vi "002 Parameter Set Control Name.vi"(8 "error in (no error)":errorcluster caption="Error In", 9 "Project":string, 10 "Read?":bool, 11 "Path In":path) -> (0 "error out":errorcluster caption="Error Out", 3 "Write":string[][](array[string]))   [LabVIEW 2020]
uses:
  0007 Controls/SY_Parameter.ctl
  Global/Data Global/Data Global Mode.ctl
  <vilib>/Utility/file.llb/Write Delimited Spreadsheet (string).vi
  <vilib>/Utility/file.llb/Read Delimited Spreadsheet (string).vi
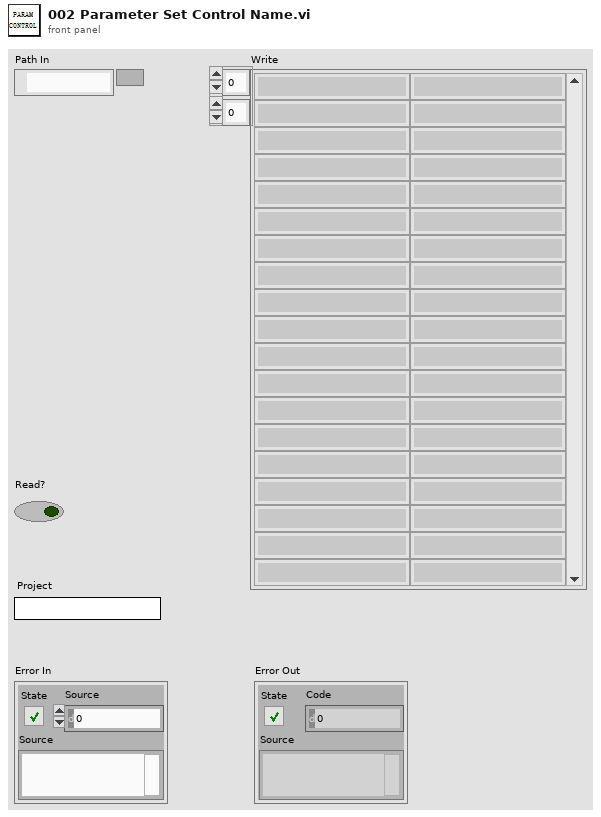
[diagram p1: front panel]
types:
  T1 = typedef "SY_Parameter.ctl" = cluster{"RH(%)":cluster{"DS":cluster{"阳极露点温度_DS":string, "阳极出口温度_DS":string, "阴极露点温度_DS":string, "阴极出口温度_DS":string, "阳极相对湿度_DS":string, "阴极相对湿度_DS":string, "阳极露点温度设置_DS":string, "阳极出口温度设置_DS":string, "阴极露点温度设置_DS":string, "阴极出口温度设置_DS":string}, "Value":cluster{"阳极露点温度_PV":sgl, "阳极出口温度_PV":sgl, "阴极露点温度_PV":sgl, "阴极出口温度_PV":sgl, "阳极相对湿度_SY":sgl, "阴极相对湿度_SY":sgl, "阳极露点温度设置_SV":sgl, "阳极出口温度设置_SV":sgl, "阴极露点温度设置_SV":sgl, "阴极出口温度设置_SV":sgl}}, "WEB":cluster{"DS":cluster{"自动模式(M0A1)_DS":string, "设备运行_DS":string, "工步号_DS":string, "运行模式_DS":string}, "Value":cluster{"自动模式(M0A1)_PV":bool, "设备运行_PV":bool, "工步号_PV":sgl, "运行模式_PV":bool}}, "ELD":cluster{"DS":cluster{"负载电压设置_DS":string, "负载电流设置_DS":string, "负载功率设置_DS":string, "负载模式设置_DS":string, "错误代码_DS":string, "负载电压_DS":string, "负载电流_DS":string, "负载功率_DS":string, "负载输出使能_DS":string, "负载连接_DS":string, "负载升压_DS":string, "负载升流_DS":string, "负载升功率_DS":string, "负载降压_DS":string, "负载降流_DS":string, "负载降功率_DS":string, "电流密度_DS":string, "功率密度_DS":string}, "Value":cluster{"负载电压设置_SV":sgl, "负载电流设置_SV":sgl, "负载功率设置_SV":sgl, "负载模式设置_SV":string, "错误代码_PV":string, "负载电压_PV":sgl, "负载电流_PV":sgl, "负载功率_PV":sgl, "负载输出使能_SV":bool, "负载连接_SY":bool, "负载升压_SV":sgl, "负载升流_SV":sgl, "负载升功率_SV":sgl, "负载降压_SV":sgl, "负载降流_SV":sgl, "负载降功率_SV":sgl, "电流密度_SV":sgl, "功率密度_SV":sgl}}, "SY":cluster{"DS":cluster{"总报警_DS":string, "WEB连接_DS":string, "计量比功能_DS":string, "PLC连接_DS":string, "H2计量比功能_DS":string, "Air计量比功能_DS":string, "PLC失联报警_DS":string}, "Value":cluster{"总报警_PV":bool, "WEB连接_PV":bool, "计量比功能_SV":bool, "PLC连接_SV":bool, "H2计量比功能_SV":bool, "Air计量比功能_SV":bool, "PLC失联报警_SV":bool}}, "PLC":cluster{"DS":cluster{"PLC急停_DS":string, "PLC连接_DS":string, "下位机心跳值_DS":string, "上位机心跳值_DS":string, "上位机报警等级字_DS":string, "负载可卸载_DS":string}, "Value":cluster{"PLC急停_PV":bool, "PLC连接_PV":bool, "下位机心跳值_PV":sgl, "上位机心跳值_SV":sgl, "上位机报警等级字_SV":sgl, "负载可卸载_SV":bool}}, "Bool Control":cluster{"DS":cluster{"维护模式_DS":string, "阳极氮气吹扫_DS":string, "阴极氮气吹扫_DS":string, "阳极脉冲使能_DS":string, "准备好使能_DS":string, "阳极干湿气切换_DS":string, "阴极干湿气切换_DS":string, "自动/手动模式_DS":string, "入口背压_DS":string, "手动卸载_DS":string, "软急停_DS":string, "负载连接_DS":string, "PLC故障复位_DS":string, "蜂鸣器屏蔽_DS":string}, "Value":cluster{"维护模式_SV":bool, "阳极氮气吹扫_SV":bool, "阴极氮气吹扫_SV":bool, "阳极脉冲使能_SV":bool, "准备好使能_SV":bool, "阳极干湿气切换_SV":bool, "阴极干湿气切换_SV":bool, "自动/手动模式_SV":bool, "入口背压_SV":bool, "手动卸载_SV":bool, "软急停_SV":bool, "负载连接_SV":bool, "PLC故障复位_SV":bool, "蜂鸣器屏蔽_SV":bool}}, "Stoich":cluster{"DS":cluster{"H2初始流量_DS":string, "Ait初始流量_DS":string, "H2侧系数_DS":string, "Air侧系数_DS":string, "H2计量比_DS":string, "Air计量比_DS":string, "时间间隔_DS":string, "H2计算气量_DS":string, "Air计算气量_DS":string, "H2流量_DS":string, "Air流量_DS":string}, "Value":cluster{"H2初始流量_SV":sgl, "Ait初始流量_SV":sgl, "H2侧系数_SV":sgl, "Air侧系数_SV":sgl, "H2计量比_SV":sgl, "Air计量比_SV":sgl, "时间间隔_SV":sgl, "H2计算气量_SV":sgl, "Air计算气量_SV":sgl, "H2流量_DS":sgl, "Air流量_DS":sgl}}, "PLC Need":cluster{"Name":string, "Identifier":string, "Source":string, "Value":string}[], "CVM":cluster{"DS":cluster{"活化面积_DS":string, "开路电压_DS":string, "单体总片数_DS":string, "单体显示片数_DS":string, "起始编号_DS":string, "最大值":string, "最大值编号_DS":string, "最小值_DS":string, "最小值编号_DS":string, "选区合计电压_DS":string, "平均值_DS":string, "离均差_DS":string}, "Value":cluster{"活化面积_SV":sgl, "开路电压_SV":sgl, "单体片数_SV":sgl, "单体显示片数_SV":sgl, "起始编号_SV":sgl, "最大值_SV":sgl, "最大值编号_SV":sgl, "最小值_SV":sgl, "最小值编号_SV":sgl, "选区合计电压_SV":sgl, "平均值_SV":sgl, "离均差_SV":sgl}}}
  T2 = typedef "Data Global Mode.ctl" = enum16{"Init", "Read", "Write", "Write Data", "Load"}
  T3 = cluster{"Name":string, "Identifier":string, "Source":string, "Value":string}[]
  T4 = cluster{"all rows[0]":string, "all rows[1]":string, "all rows[2]":string, "all rows[3]":string}
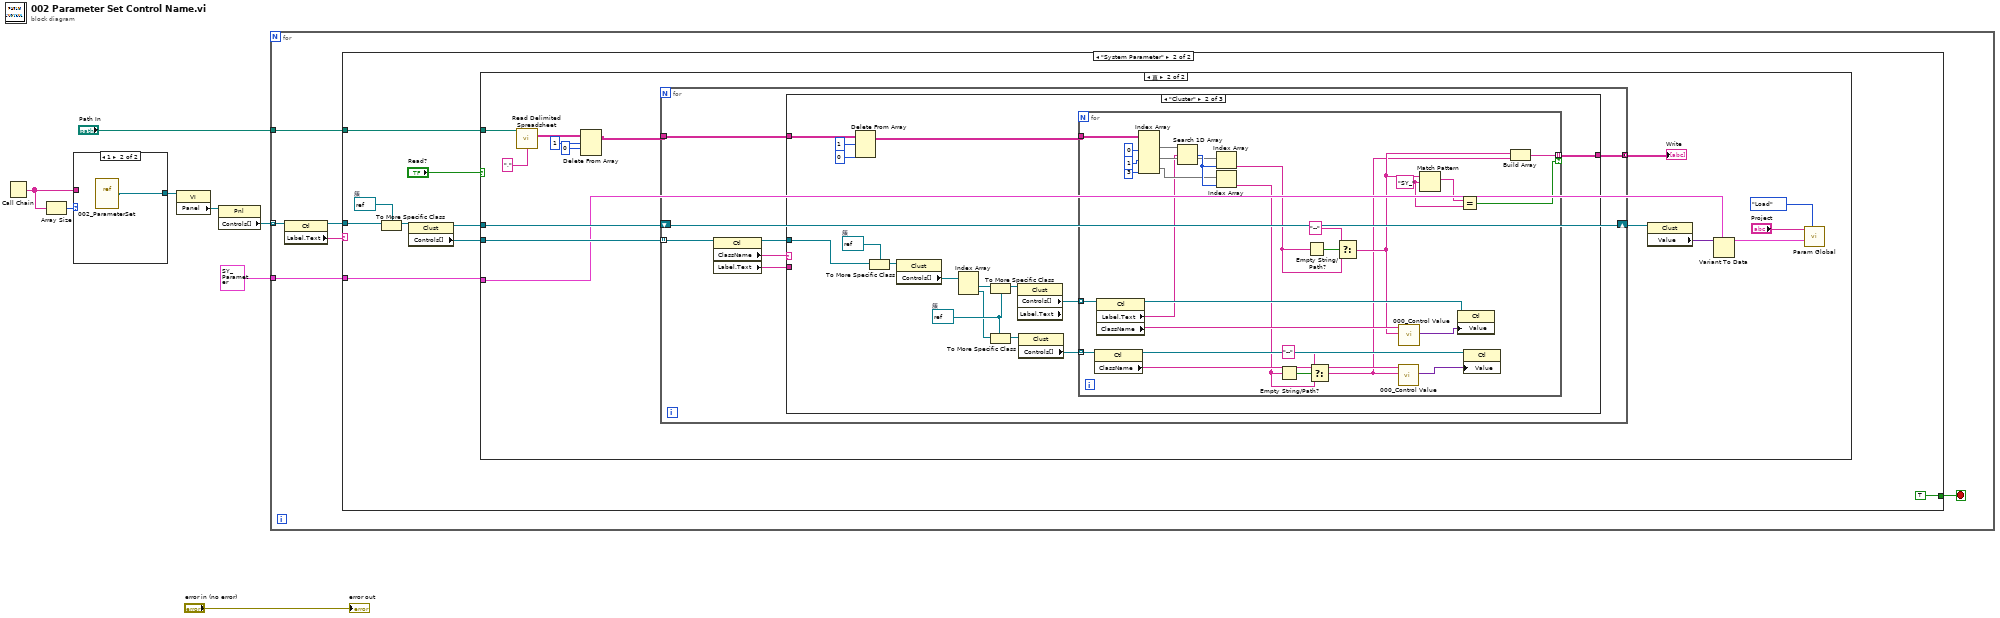
[diagram p0: block diagram]
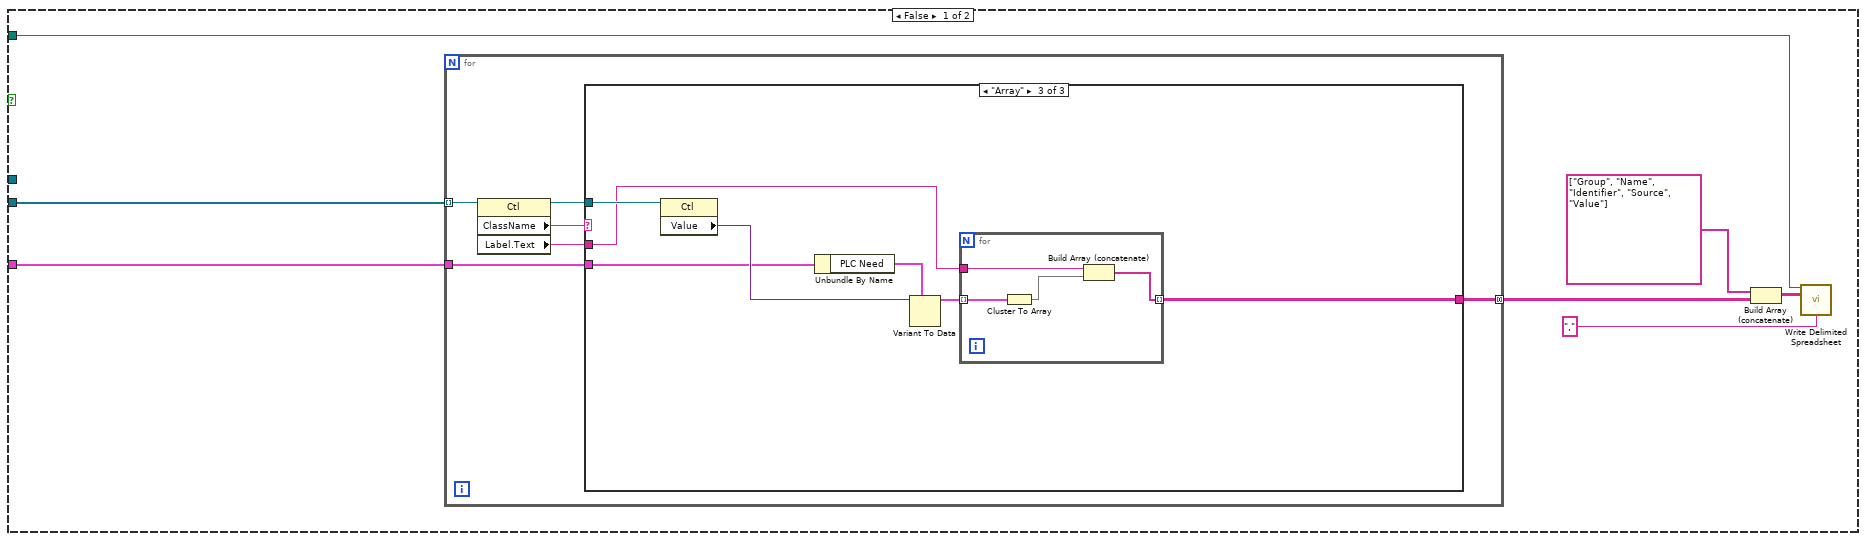
[diagram p3: hidden frame]
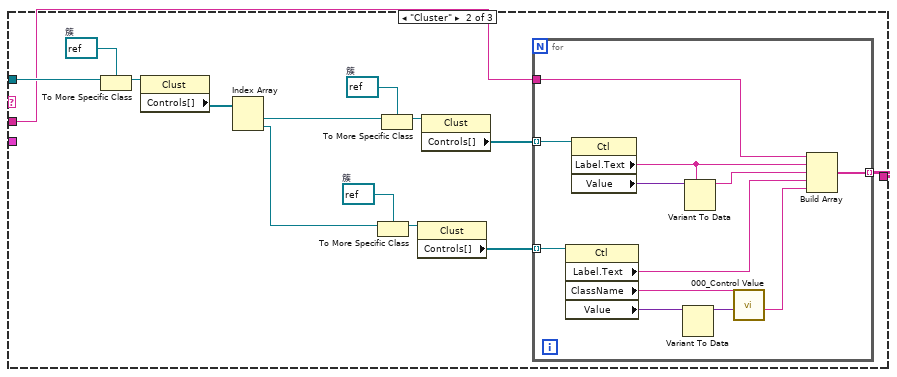
[diagram p5: hidden frame]
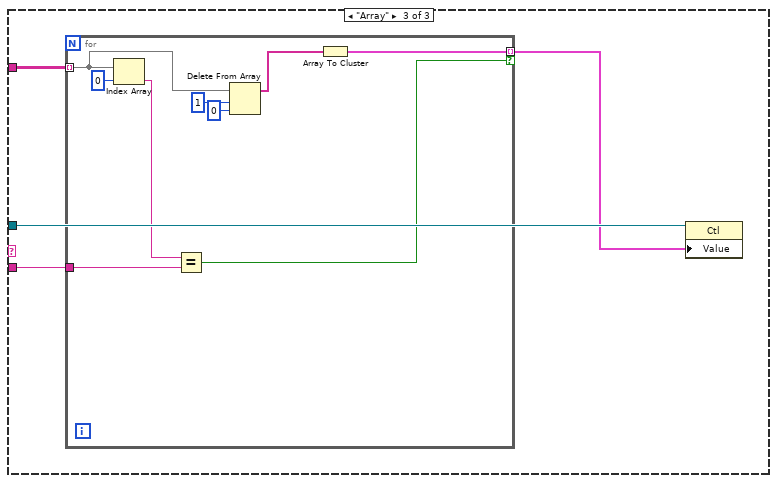
[diagram p7: hidden frame]
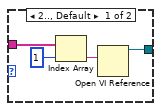
[diagram p8: hidden frame]
diagram:
  n1 = Call Chain() -> (call chain=w5:string[])
  n2 = Array Size(array=w5) -> (size(s)=w6:i32)
  n3 = case shown="1" w6 {
    tunnel: [w10 w13] -> w3
    tunnel: w5 -> [w9 _]
    frame 2.., Default {
      n4 = Index Array(array=w9, index=1 ("索引")) -> (element=w11:string)
      n5 = Open VI Reference(vi path=w11) -> (vi reference=w10:refnum<vi>)  [unwired: 5 in, 1 out]
    }
    frame 1 {
      n6 = vi-ref "002_ParameterSet.vi"() -> (w13:refnum<vi>)
    }
  }
  n7 = property class="VI"(reference=w3) -> ("Panel"=w4:refnum<vi>)  [unwired: 1 in, 2 out]
  n8 = property class="Pnl"(reference=w4) -> ("Controls[]"=w7:refnum<vi>[])  [unwired: 1 in, 2 out]
  n9 = for {
    tunnel: w7 -> [w19] mode=indexing
    tunnel: "Path In" -> [w15]
    tunnel: T1 {"RH(%)"={"DS"={"阳极露点温度_DS"="TIRC101_PV", "阳极出口温度_DS"="TIR104_PV", "阴极露点温度_DS"="TIRC301_PV", "阴极出口温度_DS"="TIRC301_PV", "阳极相对湿度_DS"="SY_RH_An", "阴极相对湿度_DS"="SY_RH_Ca", "阳极露点温度设置_DS"="TIRC101_PV", "阳极出口温度设置_DS"="TIR104_PV", "阴极露点温度设置_DS"="TIRC301_PV", "阴极出口温度设置_DS"="TIRC301_PV"}, "Value"={"阳极露点温度_PV"=0.0, "阳极出口温度_PV"=0.0, "阴极露点温度_PV"=0.0, "阴极出口温度_PV"=0.0, "阳极相对湿度_SY"=0.0, "阴极相对湿度_SY"=0.0, "阳极露点温度设置_SV"=0.0, "阳极出口温度设置_SV"=0.0, "阴极露点温度设置_SV"=0.0, "阴极出口温度设置_SV"=0.0}}, "WEB"={"DS"={"自动模式(M0A1)_DS"="AUTO_MODE", "设备运行_DS"="DEVICE_STATE", "工步号_DS"="DEVICE_STATE", "运行模式_DS"="DEVICE_STATE"}, "Value"={"自动模式(M0A1)_PV"=FALSE, "设备运行_PV"=FALSE, "工步号_PV"=0.0, "运行模式_PV"=FALSE}}, "ELD"={"DS"={"负载电压设置_DS"="EL_V_SET", "负载电流设置_DS"="EL_A_SET", "负载功率设置_DS"="EL_P_SET", "负载模式设置_DS"="EL_MODE", "错误代码_DS"="EL_ERROR", "负载电压_DS"="EL_V", "负载电流_DS"="EL_A", "负载功率_DS"="EL_P", "负载输出使能_DS"="EL_INPUT", "负载连接_DS"="ELD", "负载升压_DS"="SY_Load_Rise_Volt", "负载升流_DS"="SY_Load_Rise_Curr", "负载升功率_DS"="SY_Load_Rise_Power", "负载降压_DS"="SY_Load_Drop_Volt", "负载降流_DS"="SY_Load_Drop_Curr", "负载降功率_DS"="SY_Load_Drop_Power", "电流密度_DS"="Density_A_SV", "功率密度_DS"="Density_P_SV"}, "Value"={"负载电压设置_SV"=0.0, "负载电流设置_SV"=0.0, "负载功率设置_SV"=0.0, "负载模式设置_SV"="", "错误代码_PV"="", "负载电压_PV"=0.0, "负载电流_PV"=0.0, "负载功率_PV"=0.0, "负载输出使能_SV"=FALSE, "负载连接_SY"=FALSE, "负载升压_SV"=0.0, "负载升流_SV"=0.0, "负载升功率_SV"=0.0, "负载降压_SV"=0.0, "负载降流_SV"=0.0, "负载降功率_SV"=0.0, "电流密度_SV"=0.0, "功率密度_SV"=0.0}}, "SY"={"DS"={"总报警_DS"="SY_Totol_Warning", "WEB连接_DS"="SY_Web_Con", "计量比功能_DS"="SY_Measurung_Ratio", "PLC连接_DS"="SY_Measurung_Ratio", "H2计量比功能_DS"="SY_Measurung_Ratio", "Air计量比功能_DS"="SY_Measurung_Ratio", "PLC失联报警_DS"="SY_Measurung_Ratio"}, "Value"={"总报警_PV"=FALSE, "WEB连接_PV"=FALSE, "计量比功能_SV"=FALSE, "PLC连接_SV"=FALSE, "H2计量比功能_SV"=FALSE, "Air计量比功能_SV"=FALSE, "PLC失联报警_SV"=FALSE}}, "PLC"={"DS"={"PLC急停_DS"="HMI_Estop_SV", "PLC连接_DS"="PLC", "下位机心跳值_DS"="PLC", "上位机心跳值_DS"="HMI_AlarmWord_SV", "上位机报警等级字_DS"="HMI_AlarmWord_SV", "负载可卸载_DS"="HMI_AlarmWord_SV"}, "Value"={"PLC急停_PV"=FALSE, "PLC连接_PV"=FALSE, "下位机心跳值_PV"=0.0, "上位机心跳值_SV"=0.0, "上位机报警等级字_SV"=0.0, "负载可卸载_SV"=FALSE}}, "Bool Control"={"DS"={"维护模式_DS"="WorkMode_SV", "阳极氮气吹扫_DS"="An_Purge_SV", "阴极氮气吹扫_DS"="Ca_Purge_SV", "阳极脉冲使能_DS"="An_Pulse_EN_SV", "准备好使能_DS"="DEVICE_READY", "阳极干湿气切换_DS"="An_GasMode_SV", "阴极干湿气切换_DS"="Ca_GasMode_SV", "自动/手动模式_DS"="AUTO_MODE", "入口背压_DS"="Stack_PreMode_SV", "手动卸载_DS"="HMI_Stack_OFF_SV", "软急停_DS"="HMI_Estop_SV", "负载连接_DS"="ELoad_EN_SV", "PLC故障复位_DS"="PLC_Alarm_Reset_SV", "蜂鸣器屏蔽_DS"="BuzzerShield_SV"}, "Value"={"维护模式_SV"=FALSE, "阳极氮气吹扫_SV"=FALSE, "阴极氮气吹扫_SV"=FALSE, "阳极脉冲使能_SV"=FALSE, "准备好使能_SV"=FALSE, "阳极干湿气切换_SV"=FALSE, "阴极干湿气切换_SV"=FALSE, "自动/手动模式_SV"=FALSE, "入口背压_SV"=FALSE, "手动卸载_SV"=FALSE, "软急停_SV"=FALSE, "负载连接_SV"=FALSE, "PLC故障复位_SV"=FALSE, "蜂鸣器屏蔽_SV"=FALSE}}, "Stoich"={"DS"={"H2初始流量_DS"="SY_Activation_Area", "Ait初始流量_DS"="SY_Pieces", "H2侧系数_DS"="SY_Activation_Area", "Air侧系数_DS"="SY_Pieces", "H2计量比_DS"="SY_Activation_Area", "Air计量比_DS"="SY_Pieces", "时间间隔_DS"="SY_Stoich_Interval", "H2计算气量_DS"="SY_Stoich_H2Flow", "Air计算气量_DS"="SY_Stoich_AirFlow", "H2流量_DS"="SY_Stoich_H2Flow", "Air流量_DS"="SY_Stoich_AirFlow"}, "Value"={"H2初始流量_SV"=0.0, "Ait初始流量_SV"=0.0, "H2侧系数_SV"=0.0, "Air侧系数_SV"=0.0, "H2计量比_SV"=0.0, "Air计量比_SV"=0.0, "时间间隔_SV"=0.0, "H2计算气量_SV"=0.0, "Air计算气量_SV"=0.0, "H2流量_DS"=0.0, "Air流量_DS"=0.0}}, "PLC Need"=[], "CVM"={"DS"={"活化面积_DS"="SY_Activation_Area", "开路电压_DS"="SY_OCV_Value", "单体总片数_DS"="SY_Pieces", "单体显示片数_DS"="SY_Pieces_Dis", "起始编号_DS"="SY_Starting_Number", "最大值"="SY_Activation_Area", "最大值编号_DS"="SY_OCV_Value", "最小值_DS"="SY_Pieces", "最小值编号_DS"="SY_Pieces_Dis", "选区合计电压_DS"="SY_Starting_Number", "平均值_DS"="SY_Pieces_Dis", "离均差_DS"="SY_Starting_Number"}, "Value"={"活化面积_SV"=0.0, "开路电压_SV"=0.0, "单体片数_SV"=0.0, "单体显示片数_SV"=0.0, "起始编号_SV"=0.0, "最大值_SV"=0.0, "最大值编号_SV"=0.0, "最小值_SV"=0.0, "最小值编号_SV"=0.0, "选区合计电压_SV"=0.0, "平均值_SV"=0.0, "离均差_SV"=0.0}}} ("System Parameter") -> [w14]
    stop <- w16 stop-if-true
    n10 = property class="Ctl"(reference=w19) -> (reference out=w17:refnum<vi>, "Label.Text"=w18:string)  [unwired: 1 in, 1 out]
    n11 = case shown="\"System Parameter\"" w18 {
      tunnel: w17 -> [_ w27]
      tunnel: [_ TRUE] -> w16
      tunnel: w15 -> [_ w22]
      tunnel: w14 -> [_ w20]
      frame "eee", Default {
      }
      frame "System Parameter" {
        w26 = refnum<vi> refnum  # 簇
        n12 = To More Specific Class(target class=w26, reference=w27) -> (specific class reference=w25:refnum<vi>)  [unwired: 1 in, 1 out]
        n13 = property class="Clust"(reference=w25) -> (reference out=w21:refnum<vi>, "Controls[]"=w24:refnum<vi>[])  [unwired: 1 in, 1 out]
        n14 = case shown="真" "Read?" {
          tunnel: w24 -> [w35 w89]
          tunnel: w22 -> [w30 w93]
          tunnel: w21 -> [_ w88]
          tunnel: w20 -> [w31 w85]
          frame False {
            n15 = for {
              tunnel: w35 -> [w41] mode=indexing
              tunnel: [w37] -> w29 mode=concatenating
              tunnel: w31 -> [w36]
              n16 = property class="Ctl"(reference=w41) -> (reference out=w38:refnum<vi>, "ClassName"=w40:string, "Label.Text"=w39:string)  [unwired: 1 in, 1 out]
              n17 = case shown="\"Array\"" w40 {
                tunnel: w39 -> [_ w42 w69]
                tunnel: w38 -> [_ w54 w74]
                tunnel: [_ w51 w70] -> w37
                tunnel: w36 -> [_ _ w68]
                frame "eee", Default {
                }
                frame "Cluster" {
                  w47 = refnum<vi> refnum  # 簇
                  w49 = refnum<vi> refnum  # 簇
                  w55 = refnum<vi> refnum  # 簇
                  n18 = To More Specific Class(target class=w55, reference=w54) -> (specific class reference=w53:refnum<vi>)  [unwired: 1 in, 1 out]
                  n19 = property class="Clust"(reference=w53) -> ("Controls[]"=w52:refnum<vi>[])  [unwired: 1 in, 2 out]
                  n20 = Index Array(array=w52) -> (element #1=w48:refnum<vi>, element #2=w45:refnum<vi>)  [unwired: 2 in]
                  n21 = To More Specific Class(target class=w47, reference=w45) -> (specific class reference=w46:refnum<vi>)  [unwired: 1 in, 1 out]
                  n22 = To More Specific Class(target class=w49, reference=w48) -> (specific class reference=w50:refnum<vi>)  [unwired: 1 in, 1 out]
                  n23 = property class="Clust"(reference=w46) -> ("Controls[]"=w44:refnum<vi>[])  [unwired: 1 in, 2 out]
                  n24 = property class="Clust"(reference=w50) -> ("Controls[]"=w43:refnum<vi>[])  [unwired: 1 in, 2 out]
                  n25 = for {
                    tunnel: [w59] -> w51 mode=indexing
                    tunnel: w44 -> [w58] mode=indexing
                    tunnel: w43 -> [w57] mode=indexing
                    tunnel: w42 -> [w56]
                    n26 = property class="Ctl"(reference=w58) -> ("Label.Text"=w61:string, "ClassName"=w62:string, "Value"=w66:variant)  [unwired: 1 in, 2 out]
                    n27 = property class="Ctl"(reference=w57) -> ("Label.Text"=w65:string, "Value"=w67:variant)  [unwired: 1 in, 2 out]
                    n28 = Variant To Data(Variant=w66) -> (data=w63:variant)  [unwired: 2 in, 1 out]
                    n29 = Variant To Data(type=w65, Variant=w67) -> (data=w64:string)  [unwired: 1 in, 1 out]
                    n30 = call "000_Control Value.vi"("Value In"=w63, "Class Name"=w62) -> ("Value String Out"=w60:string)  [unwired: 8 in, 1 out]
                    n31 = Build Array(w56, w65, w64, w61, w60) -> (w59:string[])
                  }
                }
                frame "Array" {
                  n32 = property class="Ctl"(reference=w74) -> ("Value"=w72:variant)  [unwired: 1 in, 2 out]
                  n33 = Unbundle By Name(w68) -> ("PLC Need"=w73:T3)
                  n34 = Variant To Data(type=w73, Variant=w72) -> (data=w71:T3)  [unwired: 1 in, 1 out]
                  n35 = for {
                    tunnel: w71 -> [w78] mode=indexing
                    tunnel: [w76] -> w70 mode=indexing
                    tunnel: w69 -> [w75]
                    n36 = Cluster To Array(cluster=w78) -> (array=w77:string[])
                    n37 = Build Array (concatenate)(w75, w77) -> (w76:string[])
                  }
                }
              }
            }
            n38 = Build Array (concatenate)(string[] ["Group", "Name", "Identifier", "Source", "Value"], w29) -> (w33:string[][])
            n39 = call-poly <vilib>:"Write Delimited Spreadsheet.vi"("file path (dialog if empty)"=w30, "2D data"=w33, "delimiter (\\t)"="," ("delimiter (\\t)")) -> ()  [unwired: 11 in, 2 out]
          }
          frame True {
            n40 = call-poly <vilib>:"Read Delimited Spreadsheet.vi"("file path (dialog if empty)"=w93, "delimiter (\\t)"="," ("delimiter (\\t)")) -> ("all rows"=w83:string[][])  [unwired: 8 in, 5 out]
            n41 = Delete From Array(array=w83, length=1 ("长度"), index (row)=0 ("禁用的索引 (列)")) -> (array with subset deleted=w80:string[][])  [unwired: 1 in, 1 out]
            n42 = for {
              tunnel: w89 -> [w99] mode=indexing
              shift-right: [w100] -> w87
              shift-left: w88 -> [w100]
              tunnel: w80 -> [w98]
              tunnel: [w94] -> w79 mode=concatenating
              n43 = property class="Ctl"(reference=w99) -> (reference out=w97:refnum<vi>, "ClassName"=w96:string, "Label.Text"=w95:string)  [unwired: 1 in, 1 out]
              n44 = case shown="\"Cluster\"" w96 {
                tunnel: w98 -> [_ w103 w149]
                tunnel: w97 -> [_ w106 w147]
                tunnel: w95 -> [_ _ w148]
                tunnel: [_ w101 _] -> w94
                frame "eee", Default {
                }
                frame "Cluster" {
                  w109 = refnum<vi> refnum  # 簇
                  w108 = refnum<vi> refnum  # 簇
                  n45 = Delete From Array(array=w103, length=1 ("长度"), index (col)=0 ("禁用的索引 (列)")) -> (array with subset deleted=w102:string[][])  [unwired: 1 in, 1 out]
                  n46 = To More Specific Class(target class=w108, reference=w106) -> (specific class reference=w110:refnum<vi>)  [unwired: 1 in, 1 out]
                  n47 = property class="Clust"(reference=w110) -> ("Controls[]"=w111:refnum<vi>[])  [unwired: 1 in, 2 out]
                  n48 = Index Array(array=w111) -> (element #1=w115:refnum<vi>, element #2=w107:refnum<vi>)  [unwired: 2 in]
                  n49 = To More Specific Class(target class=w109, reference=w115) -> (specific class reference=w112:refnum<vi>)  [unwired: 1 in, 1 out]
                  n50 = To More Specific Class(target class=w109, reference=w107) -> (specific class reference=w114:refnum<vi>)  [unwired: 1 in, 1 out]
                  n51 = property class="Clust" props=["Controls[]", "Label", "Text"](reference=w112) -> ("Controls[]"=w113:refnum<vi>[])  [unwired: 1 in, 3 out]
                  n52 = property class="Clust"(reference=w114) -> ("Controls[]"=w116:refnum<vi>[])  [unwired: 1 in, 2 out]
                  n53 = for {
                    tunnel: w113 -> [w141] mode=indexing
                    tunnel: w116 -> [w145] mode=indexing
                    tunnel: w102 -> [w130]
                    tunnel: [w118] -> w101 mode=indexing if=w117
                    w121 = "SY_" ("正则表达式")
                    n54 = property class="Ctl"(reference=w145) -> (reference out=w143:refnum<vi>, "ClassName"=w144:string)  [unwired: 1 in, 1 out]
                    n55 = property class="Ctl"(reference=w141) -> (reference out=w138:refnum<vi>, "Label.Text"=w123:string, "ClassName"=w140:string)  [unwired: 1 in, 1 out]
                    n56 = Index Array(array=w130, index (col) #1=0 ("禁用的索引 (列)"), index (col) #2=1 ("索引 (列)"), index (col) #3=3 ("索引 (列)")) -> (element #1=w134:string[], element #2=w135:string[], element #3=w136:string[])  [unwired: 3 in]
                    n57 = Search 1D Array(1D array=w134, element=w123) -> (index of element=w137:i32)  [unwired: 1 in]
                    n58 = Index Array(array=w135, index=w137) -> (element=w124:string)
                    n59 = Index Array(array=w136, index=w137) -> (element=w127:string)
                    n60 = Empty String/Path?(string/path=w127) -> (empty?=w129:bool)
                    n61 = Empty String/Path?(string/path=w124) -> (empty?=w125:bool)
                    n62 = Select(t="--", s=w129, f=w127) -> (s? t:f=w119:string)
                    n63 = Select(t="--", s=w125, f=w124) -> (s? t:f=w120:string)
                    n64 = call "000_Control Value.vi"("Value String In"=w119, "Class Name"=w144) -> ("Value Out"=w142:variant)  [unwired: 8 in, 1 out]
                    n65 = call "000_Control Value.vi"("Value String In"=w120, "Class Name"=w140) -> ("Value Out"=w139:variant)  [unwired: 8 in, 1 out]
                    n66 = Match Pattern(string=w120, regular expression=w121) -> (match substring=w122:string)  [unwired: 1 in, 3 out]
                    n67 = property class="Ctl"(reference=w138, "Value"=w139) -> ()  [unwired: 1 in, 2 out]
                    n68 = Equal?(x=w122, y=w121) -> (x = y?=w117:bool)
                    n69 = property class="Ctl"(reference=w143, "Value"=w142) -> ()  [unwired: 1 in, 2 out]
                    n70 = Build Array(w120, w119) -> (w118:string[])
                  }
                }
                frame "Array" {
                  n71 = for {
                    tunnel: w149 -> [w154] mode=indexing
                    tunnel: w148 -> [w157]
                    tunnel: [w156] -> w146 mode=indexing if=w155
                    n72 = Index Array(array=w154, index=0 ("索引")) -> (element=w150:string)
                    n73 = Equal?(x=w150, y=w157) -> (x = y?=w155:bool)
                    n74 = Delete From Array(array=w154, length=1 ("长度"), index=0 ("索引")) -> (array with subset deleted=w151:string[])  [unwired: 1 out]
                    n75 = Array To Cluster(array=w151) -> (cluster=w156:T4)
                  }
                  n76 = property class="Ctl"(reference=w147, "Value"=w146) -> ()  [unwired: 1 in, 2 out]
                }
              }
            }
            "Write" <- w79
            n77 = property class="Clust"(reference=w87) -> ("Value"=w86:variant)  [unwired: 1 in, 2 out]
            n78 = Variant To Data(type=w85, Variant=w86) -> (data=w84:T1)  [unwired: 1 in, 1 out]
            n79 = call "Param Global.vi"("Operate"=Data_Global_Mode."Load", "Param In"=w84, "Project"="Project") -> ()  [unwired: 7 in, 2 out]
          }
        }
      }
    }
  }
  "error out" <- "error in (no error)"
